vi "Connect.vi"(8 "error in (no error)":errorcluster, 11 "Gantry in":refnum<class "A3200.lvclass">) -> (0 "error out":errorcluster, 3 "Gantry out":refnum<class "A3200.lvclass">)   [LabVIEW 2016, in "A3200.lvclass"]
uses:
  A3200.lvclass
  A3200.lvclass/A3200.ctl
  Motion.lvclass
  Drivers/Aerotech A3200/Aerotech VIs.lvlib
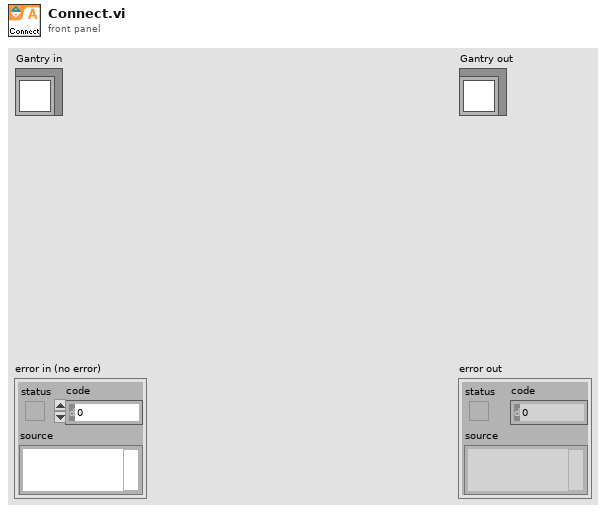
[diagram p1: front panel]
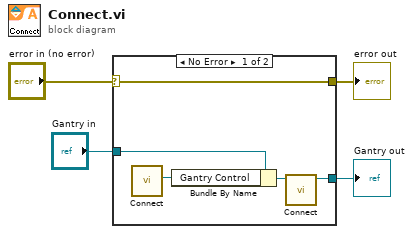
[diagram p0: block diagram]
diagram:
  n1 = case shown="No Error" "error in (no error)" {
    selector: "error in (no error)" -> [w9 w11]
    tunnel: [w9 w11] -> w3
    tunnel: [w5 w10] -> w1
    tunnel: "Gantry in" -> [w8 w10]
    frame No Error {
      n2 = call "Connect.vi"() -> ("controller"=w7:refnum<k24>)  [unwired: 10 in, 1 out]
      n3 = Bundle By Name(cluster=w8, "Gantry Control"=w7) -> (w6:refnum<class "A3200.lvclass">)
      n4 = call-parent "Connect.vi"("Motion in"=w6) -> ("Motion out"=w5:refnum<class "A3200.lvclass">)  [unwired: 9 in, 1 out]
    }
    frame Error {
    }
  }
  "error out" <- w3
  "Gantry out" <- w1
